vi "Main.vi"() -> ()   [LabVIEW 2014, in "Hello World - Multilingual Greetings (UTF-8).lvlib"]
doc: "Copyright (c) 2016 Sze Howe Koh\nThis code is licensed under the MIT license"
uses:
  Hello World - Multilingual Greetings (UTF-8).lvlib
  src/LabVIEW/LQ Core/QSize.ctl
  src/LabVIEW/Qt Widgets/QWidget/resize.vi
  src/LabVIEW/Qt Widgets/QWidget/setFont.vi
  src/LabVIEW/Qt Widgets/QWidget/setVisible.vi
  src/LabVIEW/Qt Widgets/QLabel/setText.vi
  src/LabVIEW/Qt GUI/QFont/QFont.lvclass
  src/LabVIEW/LQ Core/LQCoreEngine/LQCoreEngine.lvclass
  src/LabVIEW/Qt Widgets/QLabel/QLabel.lvclass
panel:
  in  "Greeting":string(combo)="Hello, world!"
  in  "Stop Button":bool
  # "Prerequisite knowledge/experience\n- Basic LabVIEW programming\n\n\nDescription\nThis is a \"Hello World\" app. Literally. It shows your chosen\ntranslation in a standalone label.\n\nSee the other example, \"Hello World - Introduction to Widgets\",\nfor a more comprehensive tutorial.\n\n\nShowcase\n- Displaying UTF-8 text\n- Displaying multilingual text"
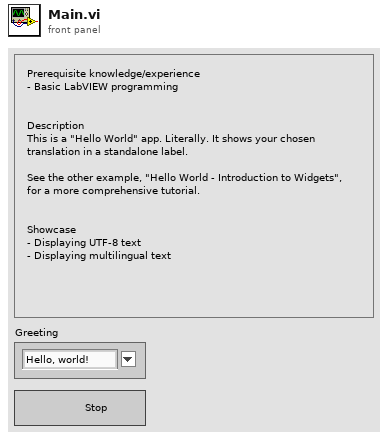
[diagram p1: front panel]
types:
  T1 = typedef "QSize.ctl" = cluster{"width":i32, "height":i32}
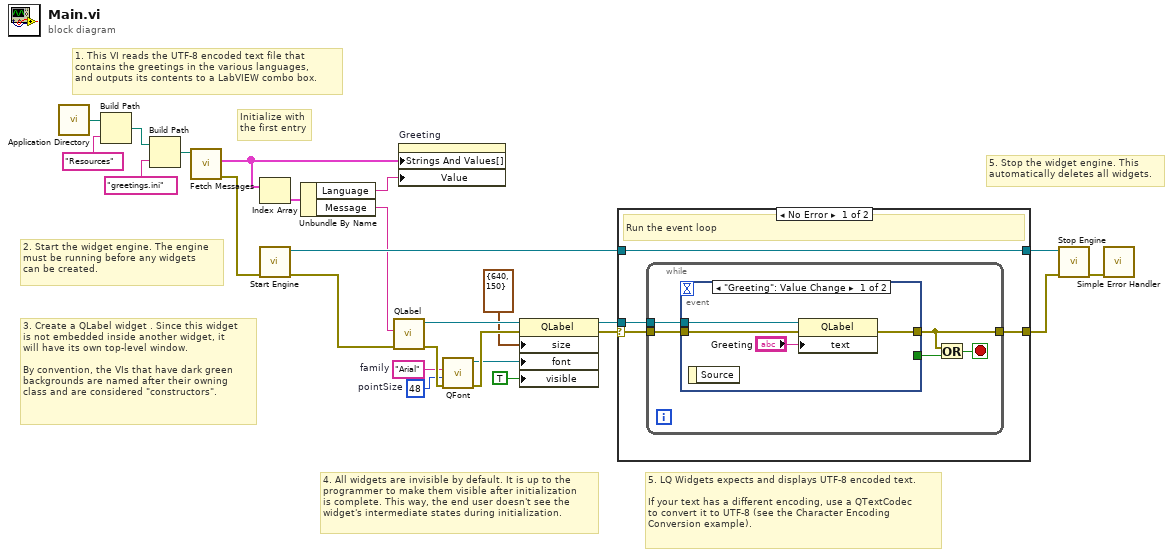
[diagram p0: block diagram]
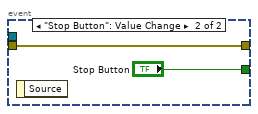
[diagram p2: hidden frame]
diagram:
  w21 = 48  # pointSize
  w22 = "Arial"  # family
  # "5. LQ Widgets expects and displays UTF-8 encoded text.\n\nIf your text has a different encoding, use a QTextCodec\nto convert it to UTF-8 (see the Character Encoding\nConversion example)."
  # "5. Stop the widget engine. This\nautomatically deletes all widgets."
  # "4. All widgets are invisible by default. It is up to the\nprogrammer to make them visible after initialization\nis complete. This way, the end user doesn't see the\nwidget's intermediate states during initialization."
  # "3. Create a QLabel widget . Since this widget\nis not embedded inside another widget, it\nwill have its own top-level window.\n\nBy convention, the VIs that have dark green\nbackgrounds are named after their owning\nclass and are considered \"constructors\"."
  # "2. Start the widget engine. The engine\nmust be running before any widgets\ncan be created."
  # "1. This VI reads the UTF-8 encoded text file that\ncontains the greetings in the various languages,\nand outputs its contents to a LabVIEW combo box."
  # "Initialize with\nthe first entry"
  n1 = call <vilib>:"Application Directory.vi"() -> ("Application Directory"=w7:path)
  n2 = Build Path(base path=w7, name or relative path="Resources") -> (appended path=w6:path)
  n3 = Build Path(base path=w6, name or relative path="greetings.ini") -> (appended path=w11:path)
  n4 = call "Fetch Messages.vi"("Greetings File Path"=w11) -> ("Error Out"=w10:errorcluster, "Greetings"=w9:cluster{"Language":string, "Message":string}[])  [unwired: 9 in]
  n5 = Index Array(array=w9) -> (element=w18:cluster{"Language":string, "Message":string})  [unwired: 1 in]
  n6 = call "Start Engine.vi"("Error In"=w10) -> ("Error Out"=w4:errorcluster, "New Engine"=w15:refnum<class "LQCoreEngine.lvclass">)  [unwired: 9 in]
  n7 = Unbundle By Name(w18) -> ("Language"=w17:string, "Message"=w5:string)
  n8 = call "QLabel.vi"("Error In"=w4, "text"=w5) -> ("Error Out"=w24:errorcluster, "New QLabel"=w20:refnum<class "QLabel.lvclass">)  [unwired: 8 in]
  n9 = property on="Greeting" class="CmbBox"("Strings And Values[]"=w9, "Value"=w17) -> ()  [unwired: 2 in, 2 out]
  n10 = call "QFont.vi"("Error In"=w24, "pointSize"=w21, "family"=w22) -> ("Error Out"=w25:errorcluster, "New QFont"=w3:refnum<class "QFont.lvclass">)  [unwired: 7 in]
  n11 = property class="QLabel"(reference=w20, error in=w25, "size"=T1 {"width"=640, "height"=150} ("minimumSize"), "font"=w3, "visible"=TRUE) -> (reference out=w23:refnum<class "QLabel.lvclass">, error out=w14:errorcluster)
  n12 = case shown="No Error" w14 {
    selector: w14 -> [w28 w41]
    tunnel: w23 -> [w29 _]
    tunnel: w15 -> [w27 w42]
    tunnel: [w27 w42] -> w13
    tunnel: [w26 w41] -> w12
    frame No Error {
      # "Run the event loop"
      n13 = while {
        tunnel: w29 -> [w34]
        tunnel: w28 -> [w33]
        tunnel: [w30] -> w26
        stop <- w32 stop-if-true
        n14 = event shown="[0] \"Greeting\": Value Change" {
          selector: _ -> [_ _]
          dyn-events: _ -> [_ _]
          timeout: _ -> [_ _]
          tunnel: w34 -> [w38 _]
          tunnel: [_ "Stop Button"] -> w31
          tunnel: w33 -> [w36 w39]
          tunnel: [w35 w39] -> w30
          event "Greeting": Value Change {
            n15 = event-data() -> ()  [unwired: 1 in, 1 out]
            n16 = property class="QLabel"(reference=w38, error in=w36, "text"="Greeting") -> (error out=w35:errorcluster)  [unwired: 1 out]
          }
          event "Stop Button": Value Change {
            n17 = event-data() -> ()  [unwired: 1 in, 1 out]
          }
        }
        n18 = Or(x=w30, y=w31) -> (x .or. y?=w32:bool)
      }
    }
    frame Error {
    }
  }
  n19 = call "Stop Engine.vi"("Error In"=w12, "LQCoreEngine"=w13) -> ("Error Out"=w1:errorcluster)  [unwired: 9 in]
  n20 = call <vilib>:"Simple Error Handler.vi"("error in (no error)"=w1) -> ()  [unwired: 4 in, 5 out]
